vi "auto avance ralentir.vi"(8 "vitesse droit":dbl, 9 "vitesse gauche":dbl, 10 "temps":dbl, 11 "temps de changement de direction":dbl) -> ()   [LabVIEW 2015]
uses:
  <vilib>/Rock Robotics/WPI/Utilities/WPI_GetSetVariantRefNum.vi
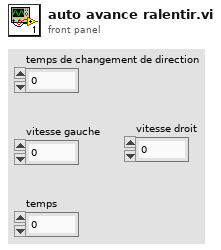
[diagram p1: front panel]
types:
  T1 = typedef "WPI_EncoderDevRef.ctl" = cluster{"DevStatus":errorcluster, "EncoderIndex":T2, "CounterIndex":T3, "DistancePerCount":dbl, "Decoding Type":T4}
  T2 = typedef "FPGA_EncoderIdx.ctl" = enum8{"Enc 0", "Enc 1", "Enc 2", "Enc 3", "Enc 4", "Enc 5", "Enc 6", "Enc 7", "Invalid"}
  T3 = typedef "FPGA_CounterCtrSystemIndex.ctl" = enum8{"Ctr 0", "Ctr 1", "Ctr 2", "Ctr 3", "Ctr 4", "Ctr 5", "Ctr 6", "Ctr 7", "Invalid"}
  T4 = typedef "WPI_EncoderType.ctl" = enum16{"1x", "2x", "4x"}
  T5 = typedef "WPI_ServoDeviceRef.ctl" = cluster{"DeviceStatus":errorcluster, "PWM Channel":T6, "DeadBand":T7}
  T6 = typedef "FPGA_DIOPWMChannel.ctl" = enum8{"PWM 0", "PWM 1", "PWM 2", "PWM 3", "PWM 4", "PWM 5", "PWM 6", "PWM 7", "PWM 8", "PWM 9", "PWM MXP 0", "PWM MXP 1", "PWM MXP 2", "PWM MXP 3", "PWM MXP 4", "PWM MXP 5", "PWM MXP 6", "PWM MXP 7", "PWM MXP 8", "PWM MXP 9", "Invalid"}
  T7 = typedef "WPI_PWMDeadband.ctl" = cluster{"Name":string, "maxPositivePwm":i32, "minPositivePwm":i32, "centerPwm":i32, "maxNegativePwm":i32, "minNegativePwm":i32, "angularRange":u16}
  T8 = typedef "WPI_RobotDriveDevRef.ctl" = cluster{"DevStatus":errorcluster, "Motors[]":T9[], "Square Inputs":bool, "Max Output":dbl}
  T9 = typedef "WPI_MotorControlDeviceRef.ctl" = cluster{"DeviceStatus":errorcluster, "Type":T10, "PWM":cluster{"PWM Channel":T6, "DeadBand":T7}, "CAN":cluster{"Device Number":u8, "Control Mode":T11, "Semaphore":T12, "Max Vout":dbl, "TalonSRX Control Mode":T13}, "Invert":bool}
  T10 = typedef "WPI_MotorControlType.ctl" = enum16{"PWM", "CAN", "CANTalonSRX"}
  T11 = typedef "WPI_CANJaguar_ControlMode.ctl" = enum8{"Percent VBus", "Current", "Speed", "Position", "Voltage"}
  T12 = typedef "Semaphore RefNum" = refnum<k1>
  T13 = typedef "WPI_CANTalonSRX_APIControlMode.ctl" = enum8{"Percent VBus", "Speed", "Position", "Slave", "Unchanged / Invalid", "Voltage Compensation", "Current", "Motion Profile"}
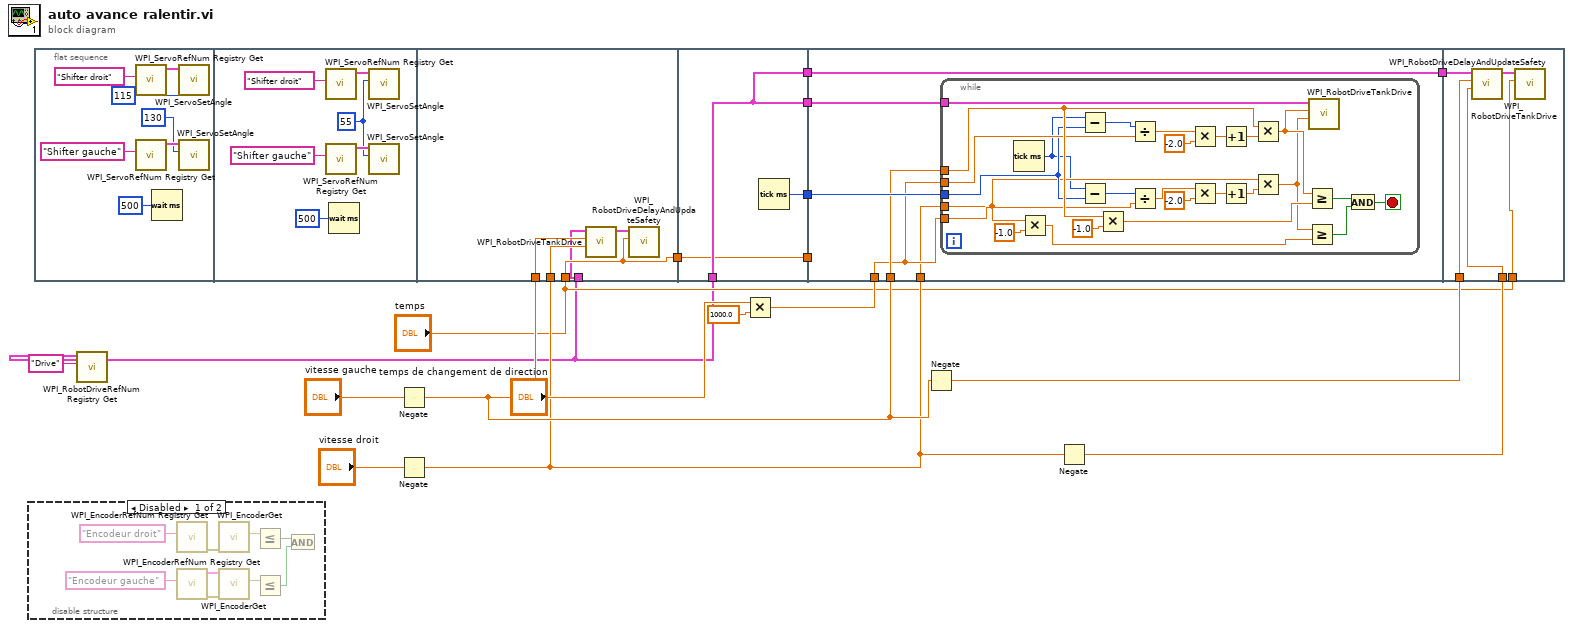
[diagram p0: block diagram]
diagram:
  n1 = disable-structure shown="Disabled" {
    frame Disabled {
      n2 = call <vilib>:"WPI_EncoderRefNum Registry Get.vi"("refnum name"="Encodeur droit") -> ("error out"=w19:errorcluster)  [unwired: 9 in, 1 out]
      n3 = call <vilib>:"WPI_EncoderRefNum Registry Get.vi"("refnum name"="Encodeur gauche") -> ("error out"=w21:errorcluster, "EncoderDevRef"=w22:T1)  [unwired: 9 in]
      n4 = call <vilib>:"WPI_EncoderGet.vi"("error in (no error)"=w19) -> ("Distance"=w24:dbl)  [unwired: 5 in, 5 out]
      n5 = call <vilib>:"WPI_EncoderGet.vi"("error in (no error)"=w21, "EncoderDevRef"=w22) -> ("Distance"=w27:dbl)  [unwired: 4 in, 5 out]
      n6 = Less Or Equal?(x=w24) -> (x <= y?=w25:bool)  [unwired: 1 in]
      n7 = Less Or Equal?(x=w27) -> (x <= y?=w26:bool)  [unwired: 1 in]
      n8 = And(x=w25, y=w26) -> ()  [unwired: 1 out]
    }
    frame Enabled {
    }
  }
  n9 = flat-sequence {
    tunnel: w6 -> [w44]
    tunnel: [w43] -> w18
    tunnel: "temps" -> [w43]
    tunnel: w4 -> [w42]
    tunnel: w1 -> [w41]
    tunnel: [w48] -> w17
    tunnel: [w47] -> w16
    tunnel: w1 -> [w47]
    tunnel: [w47] -> w15
    tunnel: w18 -> [w46]
    tunnel: [w46] -> w14
    tunnel: w17 -> [w54]
    tunnel: w16 -> [w53]
    tunnel: w15 -> [w52]
    tunnel: [w52] -> w13
    tunnel: w6 -> [w51]
    tunnel: w14 -> [_]
    tunnel: w9 -> [w50]
    tunnel: w4 -> [w49]
    tunnel: w13 -> [w84]
    tunnel: w5 -> [w83]
    tunnel: w3 -> [w82]
    tunnel: "temps" -> [w81]
    frame #0 {
      n10 = call <vilib>:"WPI_ServoRefNum Registry Get.vi"("refnum name"="Shifter droit") -> ("ServoDeviceRef"=w34:T5)  [unwired: 9 in, 1 out]
      n11 = call <vilib>:"WPI_ServoRefNum Registry Get.vi"("refnum name"="Shifter gauche") -> ("ServoDeviceRef"=w33:T5)  [unwired: 9 in, 1 out]
      n12 = Wait (ms)(milliseconds to wait=u32 500) -> ()  [unwired: 1 out]
      n13 = call <vilib>:"WPI_ServoSetAngle.vi"("Angle"=115, "ServoDeviceRef"=w34) -> ()  [unwired: 8 in, 2 out]
      n14 = call <vilib>:"WPI_ServoSetAngle.vi"("Angle"=130, "ServoDeviceRef"=w33) -> ()  [unwired: 8 in, 2 out]
    }
    frame #1 {
      w36 = 55 ("Angle")
      n15 = call <vilib>:"WPI_ServoRefNum Registry Get.vi"("refnum name"="Shifter droit") -> ("ServoDeviceRef"=w40:T5)  [unwired: 9 in, 1 out]
      n16 = call <vilib>:"WPI_ServoRefNum Registry Get.vi"("refnum name"="Shifter gauche") -> ("ServoDeviceRef"=w39:T5)  [unwired: 9 in, 1 out]
      n17 = Wait (ms)(milliseconds to wait=u32 500) -> ()  [unwired: 1 out]
      n18 = call <vilib>:"WPI_ServoSetAngle.vi"("Angle"=w36, "ServoDeviceRef"=w40) -> ()  [unwired: 8 in, 2 out]
      n19 = call <vilib>:"WPI_ServoSetAngle.vi"("Angle"=w36, "ServoDeviceRef"=w39) -> ()  [unwired: 8 in, 2 out]
    }
    frame #2 {
      n20 = call <vilib>:"WPI_RobotDriveTankDrive.vi"("Right axis value"=w42, "Left axis value"=w44, "RobotDriveDevRef"=w41) -> ("RobotDriveDevRef"=w45:T8)  [unwired: 6 in, 2 out]
      n21 = call <vilib>:"WPI_RobotDriveDelayAndUpdateSafety.vi"("Delay (s)"=w43, "RobotDriveDevRef"=w45) -> ()  [unwired: 8 in, 2 out]
    }
    frame #3 {
      n22 = Tick Count (ms)() -> (millisecond timer value=w48:u32)
    }
    frame #4 {
      n23 = while {
        tunnel: w54 -> [w59]
        tunnel: w53 -> [w60]
        tunnel: w51 -> [w79]
        tunnel: w50 -> [w76]
        tunnel: w50 -> [w58]
        tunnel: w49 -> [w57]
        stop <- w63 stop-if-true
        n24 = Tick Count (ms)() -> (millisecond timer value=w55:u32)
        n25 = Multiply(x=w57, y=-1.0) -> (x*y=w69:dbl)
        n26 = Subtract(x=w55, y=w59) -> (x-y=w75:u32)
        n27 = Subtract(x=w55, y=w59) -> (x-y=w68:u32)
        n28 = Multiply(x=w79, y=-1.0) -> (x*y=w78:dbl)
        n29 = Divide(x=w75, y=w76) -> (x/y=w73:dbl)
        n30 = Divide(x=w68, y=w58) -> (x/y=w66:dbl)
        n31 = Multiply(x=w73, y=-2.0) -> (x*y=w72:dbl)
        n32 = Multiply(x=w66, y=-2.0) -> (x*y=w65:dbl)
        n33 = Increment(x=w72) -> (x+1=w71:dbl)
        n34 = Increment(x=w65) -> (x+1=w64:dbl)
        n35 = Multiply(x=w79, y=w71) -> (x*y=w77:dbl)
        n36 = Multiply(x=w57, y=w64) -> (x*y=w56:dbl)
        n37 = Greater Or Equal?(x=w77, y=w78) -> (x >= y?=w62:bool)
        n38 = Greater Or Equal?(x=w56, y=w69) -> (x >= y?=w61:bool)
        n39 = call <vilib>:"WPI_RobotDriveTankDrive.vi"("Right axis value"=w56, "Left axis value"=w77, "RobotDriveDevRef"=w60) -> ()  [unwired: 6 in, 3 out]
        n40 = And(x=w62, y=w61) -> (x .and. y?=w63:bool)
      }
    }
    frame #5 {
      n41 = call <vilib>:"WPI_RobotDriveTankDrive.vi"("Right axis value"=w82, "Left axis value"=w83, "RobotDriveDevRef"=w84) -> ("RobotDriveDevRef"=w85:T8)  [unwired: 6 in, 2 out]
      n42 = call <vilib>:"WPI_RobotDriveDelayAndUpdateSafety.vi"("Delay (s)"=w81, "RobotDriveDevRef"=w85) -> ()  [unwired: 8 in, 2 out]
    }
  }
  n43 = call <vilib>:"WPI_RobotDriveRefNum Registry Get.vi"("refnum name"="Drive") -> ("RobotDriveDevRef"=w1:T8)  [unwired: 9 in, 1 out]
  n44 = Negate(x="vitesse gauche") -> (-x=w6:dbl)
  n45 = Negate(x="vitesse droit") -> (-x=w4:dbl)
  n46 = Multiply(x="temps de changement de direction", y=1000.0) -> (x*y=w9:dbl)
  n47 = Negate(x=w6) -> (-x=w5:dbl)
  n48 = Negate(x=w4) -> (-x=w3:dbl)
